vi "_password_db.vi"(6 "Enum":T3, 8 "Error in":errorcluster caption="Error in (no error)", 11 "Userinfo":T1) -> (0 "Error out":errorcluster, 2 "Boolean":bool, 3 "Userinfo (dup)":T1)   [LabVIEW 2020]
uses:
  Typedef/User-Info.ctl
  Typedef/User-Role.ctl
  _password_db_oper.ctl
panel:
  out "appended array":T1[](array[typedef])
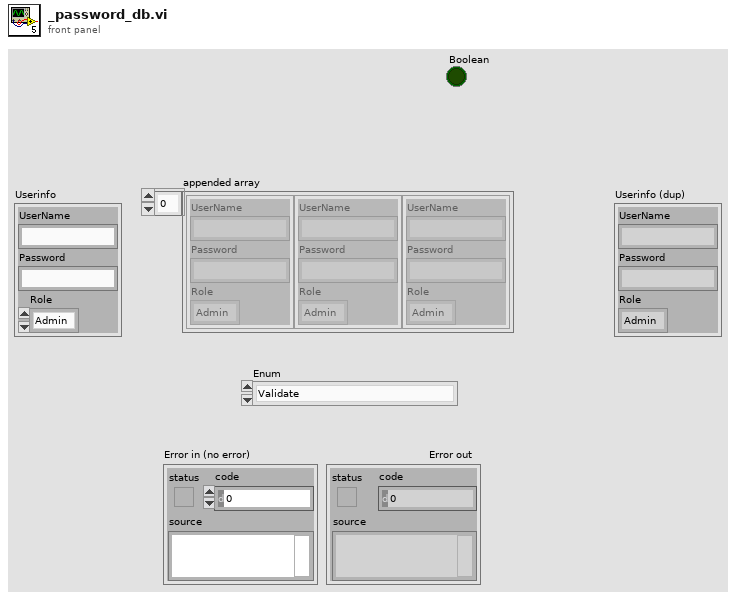
[diagram p1: front panel]
types:
  T1 = typedef "User-Info.ctl" = cluster{"UserName":string, "Password":string, "Role":T2}
  T2 = typedef "User-Role.ctl" = enum16{"Admin", "Engineer", "Operator"}
  T3 = typedef "_password_db_oper.ctl" = enum16{"Validate", "Register", "Unregister", "View"}
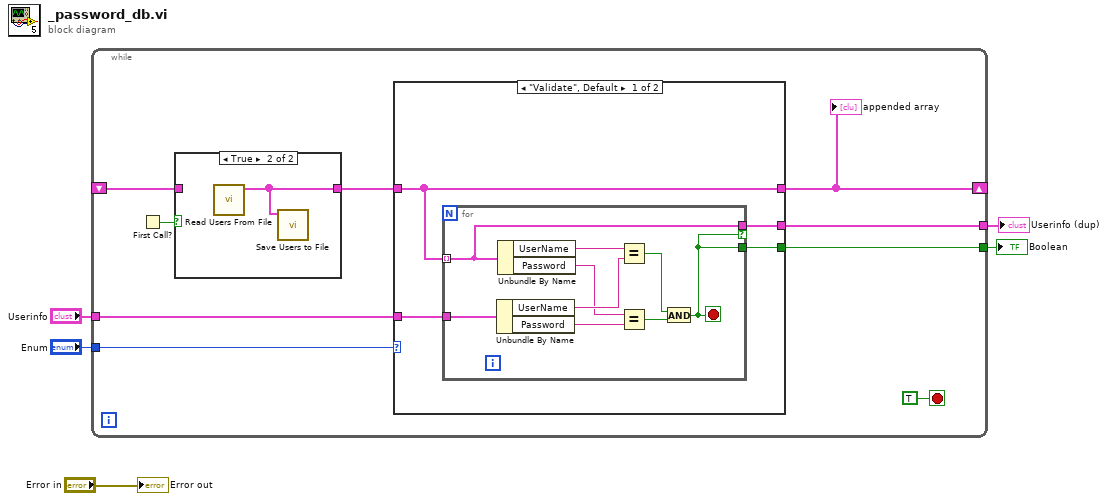
[diagram p0: block diagram]
diagram:
  n1 = while {
    shift-right: [w10] -> _
    shift-left: _ -> [w11]
    tunnel: "Enum" -> [w9]
    tunnel: "Userinfo" -> [w8]
    tunnel: [w7] -> w2
    tunnel: [w6] -> w1
    stop <- TRUE stop-if-true
    n2 = First Call?() -> (First Call?: T/F=w12:bool)
    n3 = case shown="True" w12 {
      tunnel: [w15 w16] -> w13
      tunnel: w11 -> [w15 _]
      frame False {
      }
      frame True {
        n4 = call "Read Users From File.vi"() -> ("Array"=w16:T1[])  [unwired: 10 in, 1 out]
        n5 = call "Save Users to File.vi"("Array"=w16) -> ()  [unwired: 10 in, 1 out]
      }
    }
    n6 = case shown="\"Validate\", Default" w9 {
      tunnel: [w20 w30] -> w10
      tunnel: w13 -> [w20 w30]
      tunnel: w8 -> [w19 _]
      tunnel: [w18 _] -> w7
      tunnel: [w17 _] -> w6
      frame "Validate", Default {
        n7 = for {
          tunnel: w20 -> [w22] mode=indexing
          tunnel: w19 -> [w29]
          tunnel: [w21] -> w18
          tunnel: [w22] -> w17 if=w21
          stop <- w21 stop-if-true
          n8 = Unbundle By Name(w29) -> ("UserName"=w27:string, "Password"=w26:string)
          n9 = Unbundle By Name(w22) -> ("UserName"=w28:string, "Password"=w25:string)
          n10 = Equal?(x=w28, y=w27) -> (x = y?=w23:bool)
          n11 = Equal?(x=w25, y=w26) -> (x = y?=w24:bool)
          n12 = And(x=w23, y=w24) -> (x .and. y?=w21:bool)
        }
      }
      frame "Register" {
      }
    }
    "appended array" <- w10
  }
  "Boolean" <- w2
  "Userinfo (dup)" <- w1
  "Error out" <- "Error in"
